vi "20211008_HW01.vi"() -> ()   [LabVIEW 2019]
panel:
  out "Number of True":i32
  in  "Array":bool[](array[boolean])
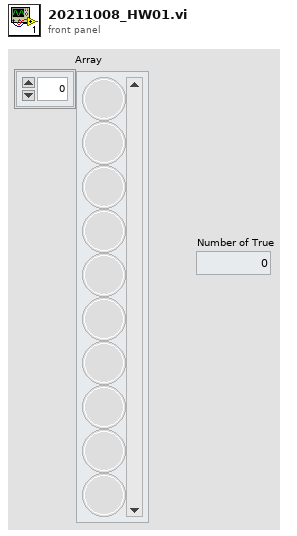
[diagram p1: front panel]
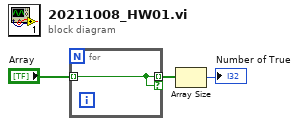
[diagram p0: block diagram]
diagram:
  n1 = for {
    tunnel: "Array" -> [w4] mode=indexing
    tunnel: [w4] -> w2 mode=indexing if=w4
  }
  n2 = Array Size(array=w2) -> (size(s)=→"Number of True":i32)
